vi "Filter select.vi"(1 "Filter:":u16(ring) items=["No filter", "100 nm Al", "200 nm Al", "250 nm Al", "500 nm Al"]) -> (0 "filter data":cluster{"Numeric":dbl, dbl}[](array[cluster]))   [LabVIEW 2019]
uses:
  <vilib>/Utility/file.llb/Read Delimited Spreadsheet (DBL).vi
panel:
  out "XY Graph":cluster{"X":dbl, "Y":dbl}[](graph)
  in  "file path for tab delimited 500nm Al text file":path=path "C:/Users/Spenser Burrows/Desktop/Work/Labview software for spectrometer/500nmAl.txt"
  in  "file path for tab delimited 250nm Al text file":path=path "C:/Users/Spenser Burrows/Desktop/Work/Labview software for spectrometer/250nmAl.txt"
  in  "file path for tab delimited 200nm Al text file":path=path "C:/Users/Spenser Burrows/Desktop/Work/Labview software for spectrometer/200nmAl.txt"
  out "Transmission":dbl[](array[numeric])
  out "eV":dbl[](array[numeric])
  in  "file path for tab delimited 100nm Al text file":path=path "C:/Users/Spenser Burrows/Desktop/Work/Labview software for spectrometer/100nmAl.txt"
  # "Find appopriate filter .txt file on the machine that this vi is being run on, then right click on the file box, go to data operations, and make current value default"
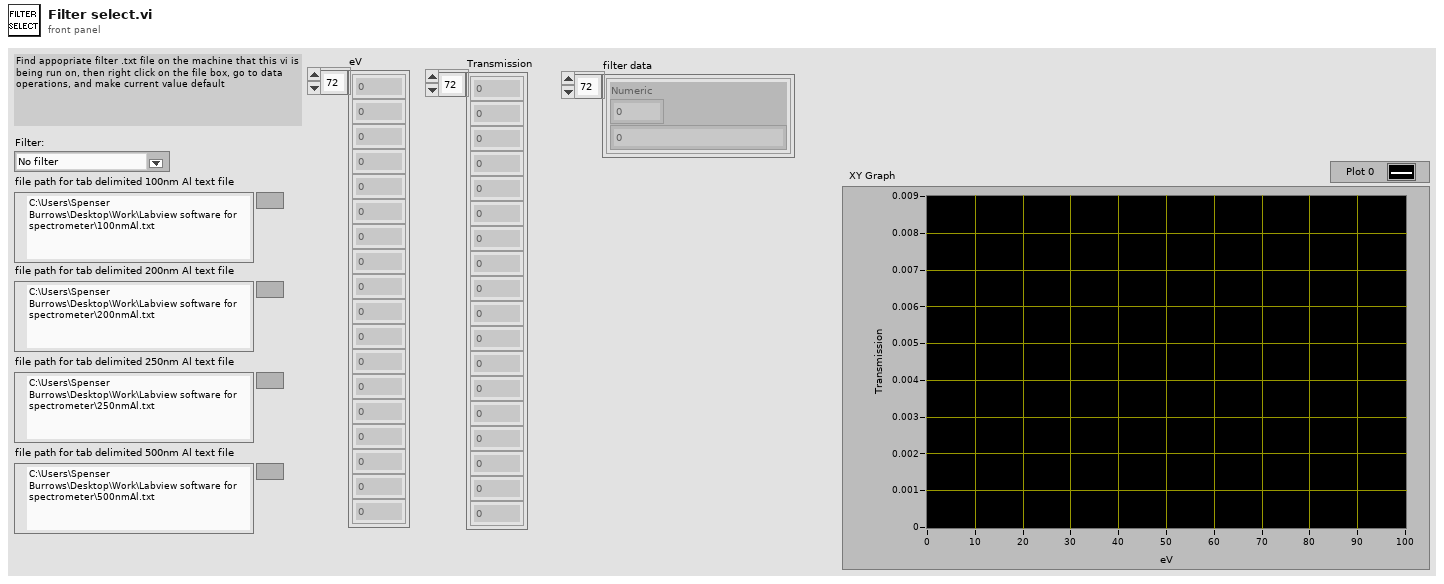
[diagram p1: front panel]
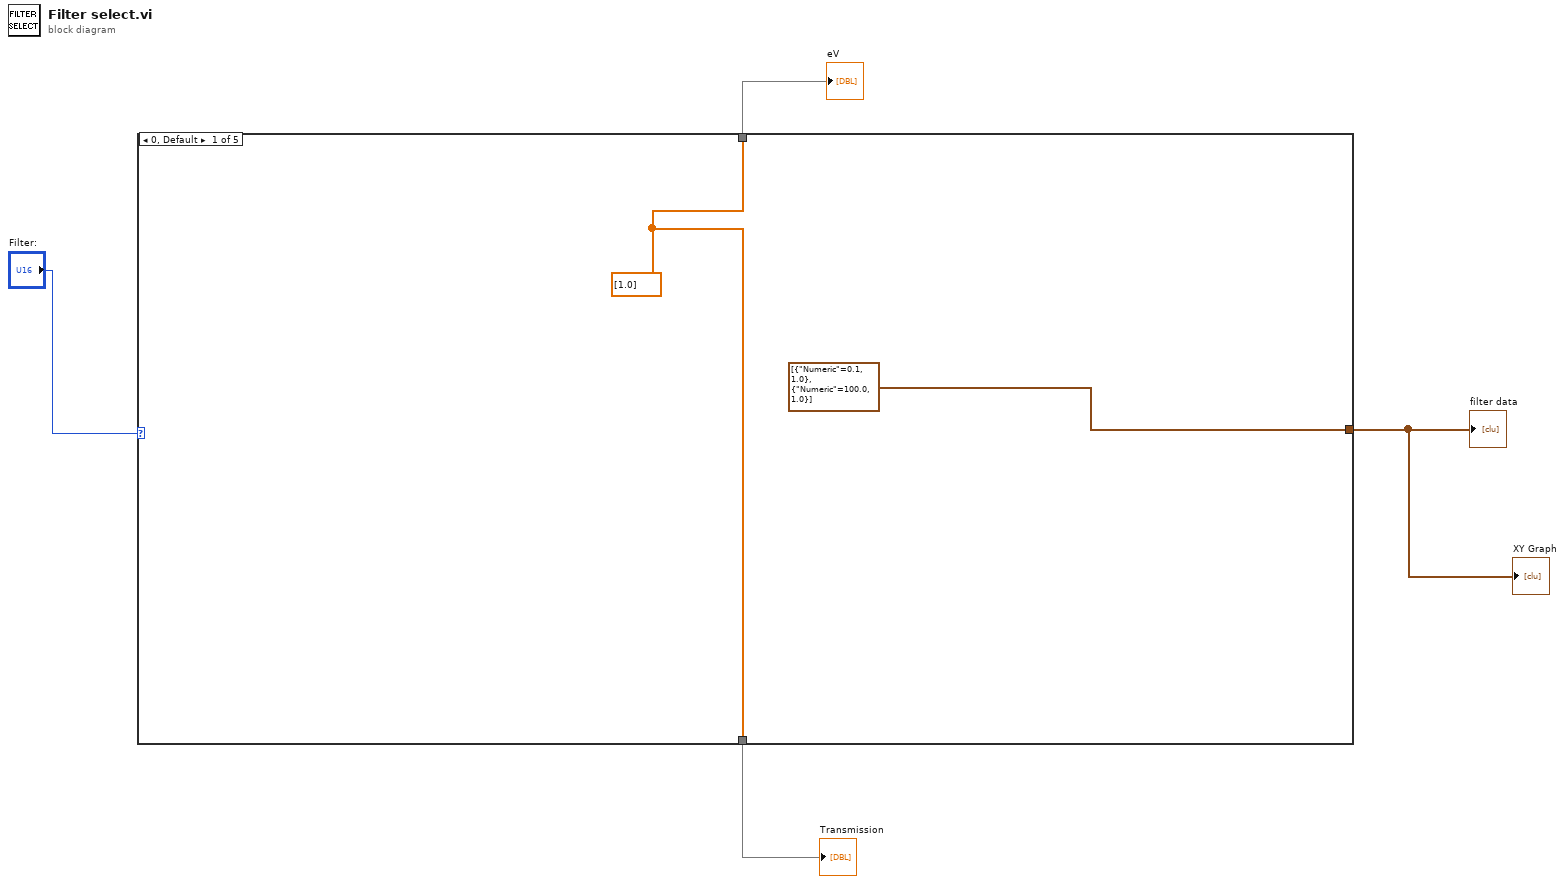
[diagram p0: block diagram]
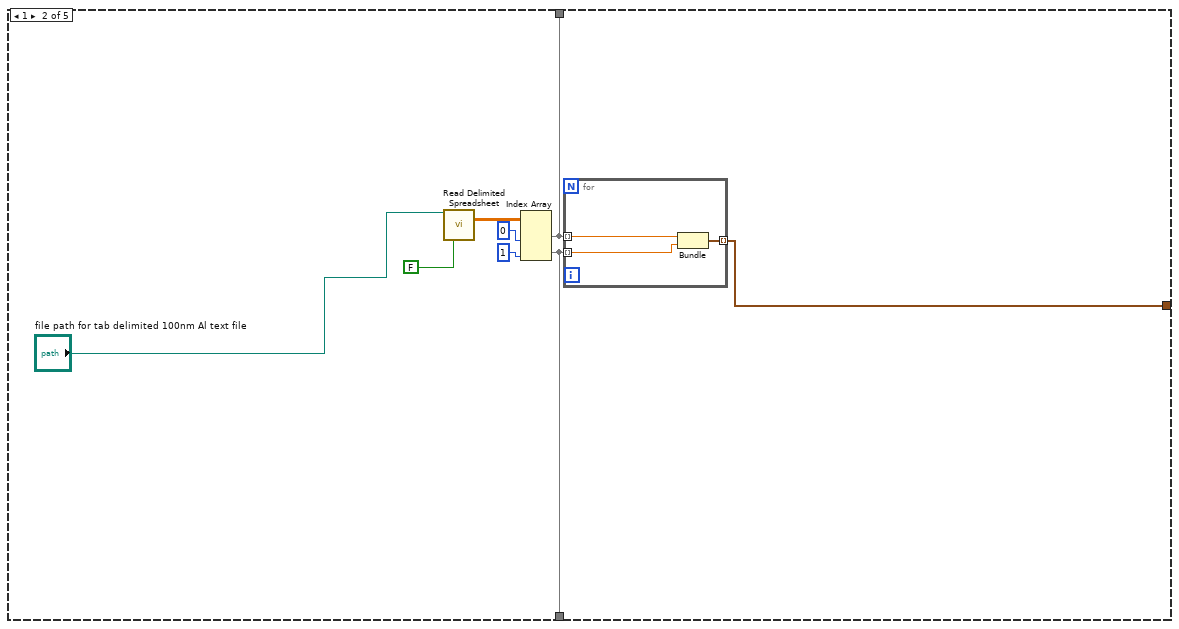
[diagram p2: hidden frame]
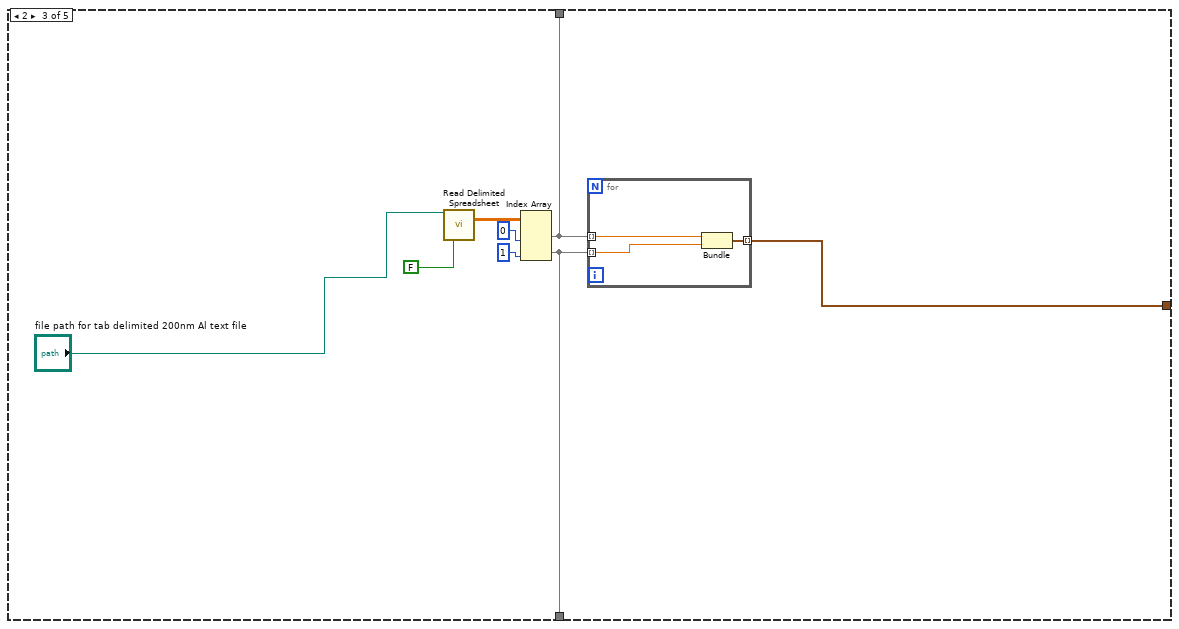
[diagram p3: hidden frame]
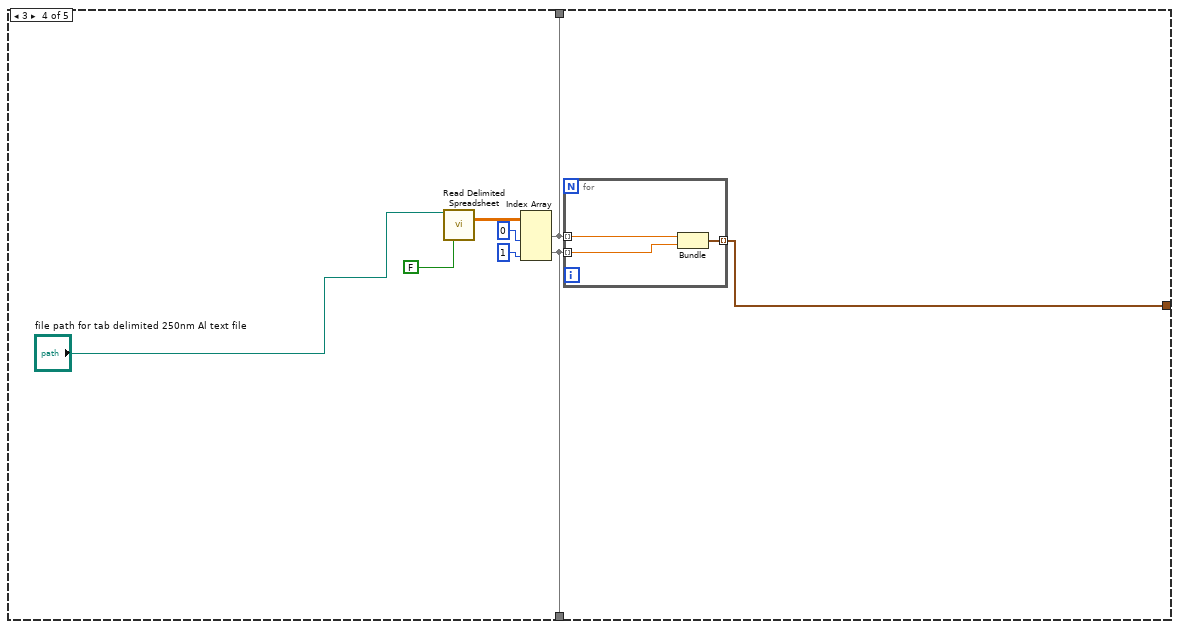
[diagram p4: hidden frame]
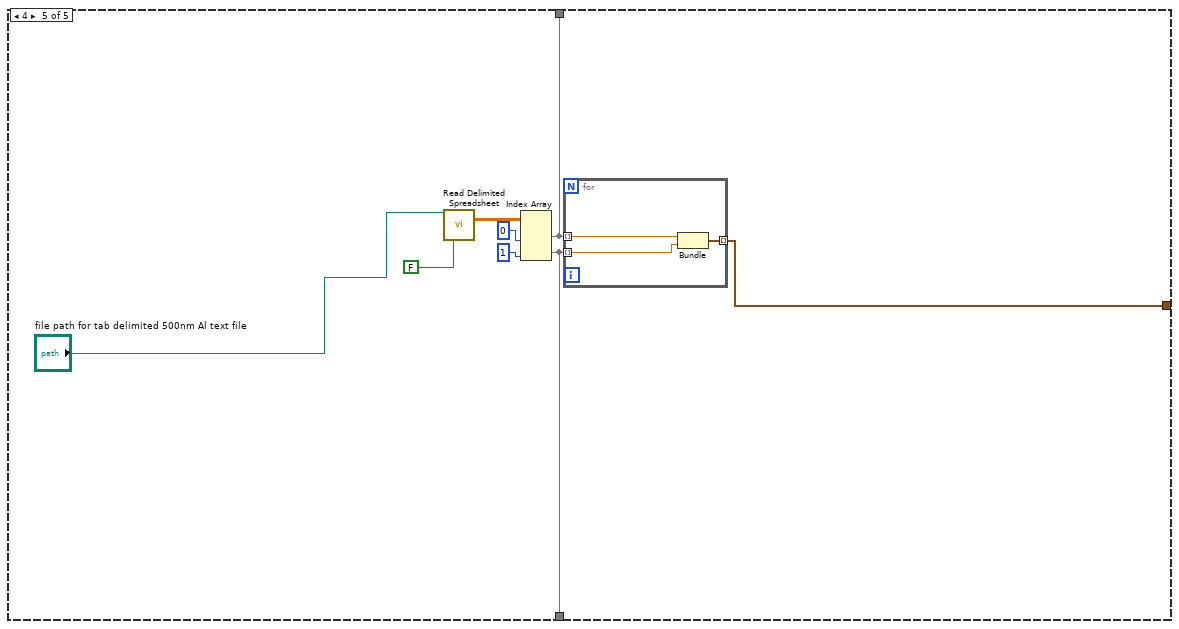
[diagram p5: hidden frame]
diagram:
  n1 = case shown="0, Default" "Filter:" {
    tunnel: [cluster{"Numeric":dbl, dbl}[] [{"Numeric"=0.1, 1.0}, {"Numeric"=100.0, 1.0}] w9 w18 w31 w42] -> w1
    tunnel: [w5 w8 w20 w30 w41] -> w3
    tunnel: [w5 w7 w19 w29 w40] -> w2
    frame 0, Default {
      w5 = dbl[] [1.0] ("all rows")
    }
    frame 1 {
      n2 = call-poly <vilib>:"Read Delimited Spreadsheet.vi"("file path (dialog if empty)"="file path for tab delimited 100nm Al text file", "transpose? (F)"=FALSE) -> ("all rows"=w11:dbl[][])  [unwired: 8 in, 5 out]
      n3 = Index Array(array=w11, index (col) #1=0 ("disabled index (col)"), index (col) #2=1 ("disabled index (col)")) -> (element #1=w8:dbl[], element #2=w7:dbl[])  [unwired: 2 in]
      n4 = for {
        tunnel: w8 -> [w17] mode=indexing
        tunnel: w7 -> [w15] mode=indexing
        tunnel: [w16] -> w9 mode=indexing
        n5 = Bundle("Numeric"=w17, "Numeric"=w15) -> (w16:cluster{"Numeric":dbl, "Numeric":dbl})  [unwired: 1 in]
      }
    }
    frame 2 {
      n6 = call-poly <vilib>:"Read Delimited Spreadsheet.vi"("file path (dialog if empty)"="file path for tab delimited 200nm Al text file", "transpose? (F)"=FALSE) -> ("all rows"=w22:dbl[][])  [unwired: 8 in, 5 out]
      n7 = Index Array(array=w22, index (col) #1=0 ("disabled index (col)"), index (col) #2=1 ("disabled index (col)")) -> (element #1=w20:dbl[], element #2=w19:dbl[])  [unwired: 2 in]
      n8 = for {
        tunnel: w20 -> [w28] mode=indexing
        tunnel: w19 -> [w26] mode=indexing
        tunnel: [w27] -> w18 mode=indexing
        n9 = Bundle("Numeric"=w28, "Numeric"=w26) -> (w27:cluster{"Numeric":dbl, "Numeric":dbl})  [unwired: 1 in]
      }
    }
    frame 3 {
      n10 = call-poly <vilib>:"Read Delimited Spreadsheet.vi"("file path (dialog if empty)"="file path for tab delimited 250nm Al text file", "transpose? (F)"=FALSE) -> ("all rows"=w33:dbl[][])  [unwired: 8 in, 5 out]
      n11 = Index Array(array=w33, index (col) #1=0 ("disabled index (col)"), index (col) #2=1 ("disabled index (col)")) -> (element #1=w30:dbl[], element #2=w29:dbl[])  [unwired: 2 in]
      n12 = for {
        tunnel: w30 -> [w39] mode=indexing
        tunnel: w29 -> [w37] mode=indexing
        tunnel: [w38] -> w31 mode=indexing
        n13 = Bundle("Numeric"=w39, "Numeric"=w37) -> (w38:cluster{"Numeric":dbl, "Numeric":dbl})  [unwired: 1 in]
      }
    }
    frame 4 {
      n14 = call-poly <vilib>:"Read Delimited Spreadsheet.vi"("file path (dialog if empty)"="file path for tab delimited 500nm Al text file", "transpose? (F)"=FALSE) -> ("all rows"=w44:dbl[][])  [unwired: 8 in, 5 out]
      n15 = Index Array(array=w44, index (col) #1=0 ("disabled index (col)"), index (col) #2=1 ("disabled index (col)")) -> (element #1=w41:dbl[], element #2=w40:dbl[])  [unwired: 2 in]
      n16 = for {
        tunnel: w41 -> [w50] mode=indexing
        tunnel: w40 -> [w48] mode=indexing
        tunnel: [w49] -> w42 mode=indexing
        n17 = Bundle("Numeric"=w50, "Numeric"=w48) -> (w49:cluster{"Numeric":dbl, "Numeric":dbl})  [unwired: 1 in]
      }
    }
  }
  "filter data" <- w1
  "eV" <- w3
  "Transmission" <- w2
  "XY Graph" <- w1
